vi "laneleftright.vi"() -> (2 "Coeff right":dbl[](array[numeric]), 3 "Coeff left":dbl[](array[numeric]))   [LabVIEW 2015]
uses:
  G_LCM.vi
  G_SEN.vi
  <vilib>/Analysis/1siggen.llb/Ramp Pattern by Delta.vi
  <vilib>/Analysis/polynomials.llb/1D Polynomial Evaluation (DBL).vi
  <vilib>/Analysis/NI_AALPro.lvlib
  <vilib>/Analysis/NI_AALBase.lvlib
panel:
  out "c_tmp":dbl[](array[numeric])
  out "y_tmp":dbl[](array[numeric])
  out "x_tmp":dbl[](array[numeric])
  out "Boolean":bool
  out "y origin":dbl[](array[numeric])
  out "x origin":dbl[](array[numeric])
  out "Histogram Graph 2":T1(graph)
  out "right":dbl[](graph)
  out "left":dbl[](graph)
  in  "Numeric":i32=4
  out "error left":dbl[](array[numeric])
  out "error right":dbl[](array[numeric])
  out "y seed":dbl[](array[numeric])
  out "XY Graph 4":cluster{"Y":dbl[], "Y":dbl[]}[](graph)=[{"Y"=array[3210 elements], "Y"=array[3210 elements]}, {"Y"=[-0.0, 0.001154394197769193, 0.004617650635850623, 0.010389990872226917, 0.018471784248973222, 0.02886354801042046, 0.041565947468740205, 0.056579796217107514, 0.0739060563904701, 0.0935458389742223, 0.11550040416098284, 0.13977116175580306, 0.16635967162997645, 0.19526764422393228, 0.2264969410994837, 0.26004957554195585, 0.2959277132125635, 0.3341336728515216, 0.374669927032528, 0.417539102969144, 0.4627439833735707, 0.5102875073687159, 0.560172771454063, 0.6124030305261954, 0.6669816989546717, 0.7239123517142048, 0.7831987255740245, 0.8448447203451934, 0.9088544001870815, 0.975231994973953, 1.0439819017227023, 1.1151086860829622, 1.1886170838907617, 1.2645120027869723, 1.342798523901962, 1.42348190360768, 1.5065675753387922, 1.592061151484188, 1.6799684253507792, 1.770295373200753, 1.8630481563645134, 1.9582331234307588, 2.0558568125157564, 2.1559259536137603, 2.258447471030621], "Y"=[0.0, 0.5, 1.0, 1.5, 2.0, 2.5, 3.0, 3.5, 4.0, 4.5, 5.0, 5.5, 6.0, 6.5, 7.0, 7.5, 8.0, 8.5, 9.0, 9.5, 10.0, 10.5, 11.0, 11.5, 12.0, 12.5, 13.0, 13.5, 14.0, 14.5, 15.0, 15.5, 16.0, 16.5, 17.0, 17.5, 18.0, 18.5, 19.0, 19.5, 20.0, 20.5, 21.0, 21.5, 22.0]}, {"Y"=[0.362252581831572], "Y"=[-0.8199241909738847]}, {"Y"=array[210 elements], "Y"=array[210 elements]}, {"Y"=[-0.925, -0.925, -0.925, -0.6775, -0.6775, -0.925, -0.925, -0.925, -0.925, -0.6775, -0.6775, -0.925, -0.925, -0.925, 0.9025, 0.9025, 0.9025, 0.6775, 0.6775, 0.9025, 0.9025, 0.9025, 0.9025, 0.6775, 0.6775, 0.9025, 0.9025, 0.9025, -0.925], "Y"=[-0.75, -0.224, 0.224, 0.224, -0.224, -0.224, 0.224, 2.415, 2.885, 2.885, 2.415, 2.415, 2.885, 3.5, 3.5, 2.885, 2.415, 2.415, 2.885, 2.885, 2.415, 0.224, -0.224, -0.224, 0.224, 0.224, -0.224, -0.75, -0.75]}, {"Y"=[0.171875, 0.15377271904051304, 0.1346290179491043, 0.11445423440635205, 0.09325870609283447, 0.07105277068912982, 0.04784676587581635, 0.02365102933347224, -0.0015241012573242174, -0.02766828821599482, -0.05477119386196136, -0.08282248051464558, -0.11181181049346922, -0.14172884611785413, -0.17256324970722198, -0.20430468358099463, -0.23694281005859374, -0.27046729145944115, -0.30486779010295867, -0.340133968308568, -0.3762554883956909, -0.41322201268374914, -0.4510232034921646, -0.4896487231403589], "Y"=[0.0, 0.5, 1.0, 1.5, 2.0, 2.5, 3.0, 3.5, 4.0, 4.5, 5.0, 5.5, 6.0, 6.5, 7.0, 7.5, 8.0, 8.5, 9.0, 9.5, 10.0, 10.5, 11.0, 11.5]}, {"Y"=[1.796875, 1.778772719040513, 1.7596290179491043, 1.739454234406352, 1.7182587060928345, 1.6960527706891297, 1.6728467658758164, 1.6486510293334722, 1.6234758987426758, 1.5973317117840051, 1.5702288061380387, 1.5421775194853544, 1.513188189506531, 1.483271153882146, 1.452436750292778, 1.4206953164190055, 1.3880571899414063, 1.354532708540559, 1.3201322098970414, 1.284866031691432, 1.248744511604309, 1.2117779873162509, 1.1739767965078354, 1.135351276859641, 1.0959117660522462, 1.0556686017662287, 1.014632121682167, 0.9728126634806396, 0.9302205648422242, 0.8868661634474992], "Y"=[0.0, 0.5, 1.0, 1.5, 2.0, 2.5, 3.0, 3.5, 4.0, 4.5, 5.0, 5.5, 6.0, 6.5, 7.0, 7.5, 8.0, 8.5, 9.0, 9.5, 10.0, 10.5, 11.0, 11.5, 12.0, 12.5, 13.0, 13.5, 14.0, 14.5]}, {"Y"=[-1.453125, -1.471227280959487, -1.4903709820508957, -1.510545765593648, -1.5317412939071655, -1.5539472293108703, -1.5771532341241836, -1.6013489706665278, -1.6265241012573242, -1.6526682882159949, -1.6797711938619613, -1.7078224805146456, -1.736811810493469, -1.766728846117854, -1.797563249707222, -1.8293046835809945, -1.8619428100585937, -1.895467291459441, -1.9298677901029586], "Y"=[0.0, 0.5, 1.0, 1.5, 2.0, 2.5, 3.0, 3.5, 4.0, 4.5, 5.0, 5.5, 6.0, 6.5, 7.0, 7.5, 8.0, 8.5, 9.0]}, {"Y"=[0.171875, 0.2568230007600336, 0.3384052130063493, 0.44574342526006827, 0.5205081969556753, 0.5917680690742042, 0.659409530134929, 0.7229937549325056, 0.7835496148685115, 0.8405449546633443, 0.9258576868463875], "Y"=[-20.239964538708662, -19.725637940364884, -19.211158961966362, -18.6998967366845, -18.19022720070031, -17.681887266143153, -17.17615515566314, -16.67683575591291, -16.176265245349786, -15.679082775270938, -15.183754484614711]}, {"Y"=[7.134647485270904], "Y"=[38.71960961082238]}, {"Y"=array[980 elements], "Y"=array[980 elements]}, {"Y"=[], "Y"=[]}]
  out "y all":dbl[](array[numeric])
  out "x all":dbl[](array[numeric])
  out "x_left":dbl[](array[numeric])
  out "x_right":dbl[](array[numeric])
  out "y_left":dbl[](array[numeric])
  out "y_right":dbl[](array[numeric])
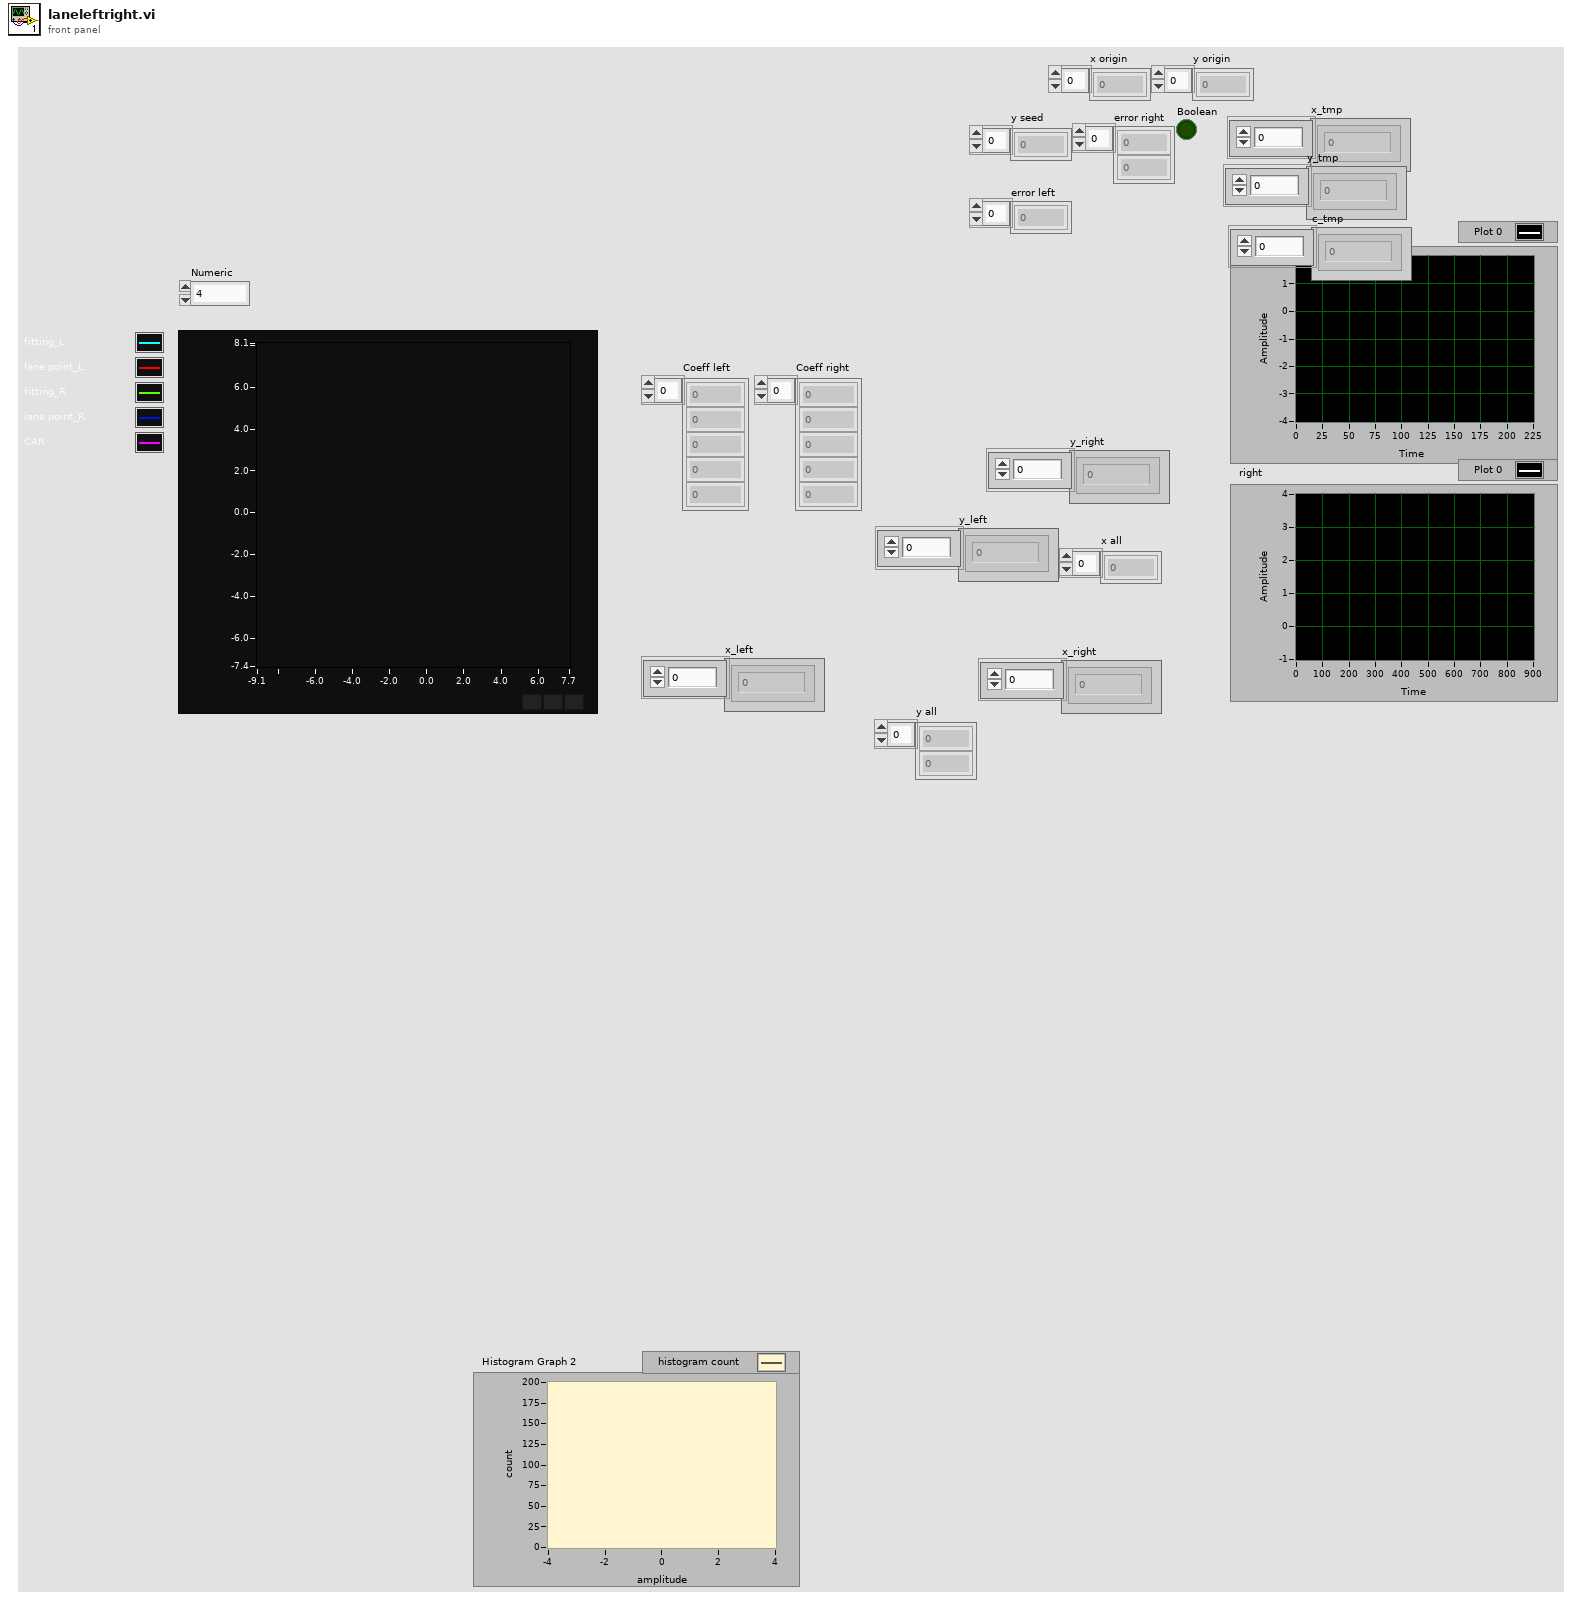
[diagram p1: front panel]
types:
  T1 = cluster{"X Values":dbl[], "Histogram: h(x)":i32[]}
  T2 = cluster{"hash":i64, "sys time":i64, "size":i64, "x":dbl[], "y":dbl[]}
  T3 = cluster{"delta":bool, "Rotational position":dbl, "Rotational position":dbl}[]
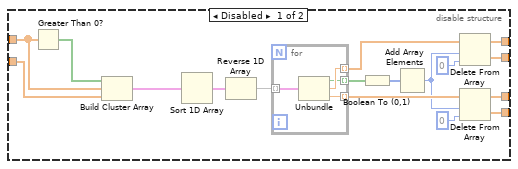
[diagram p3: hidden frame]
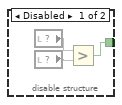
[diagram p6: hidden frame]
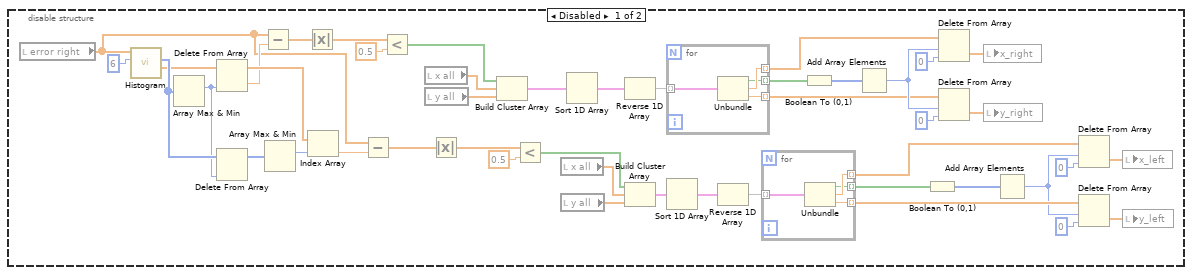
[diagram p7: hidden frame]
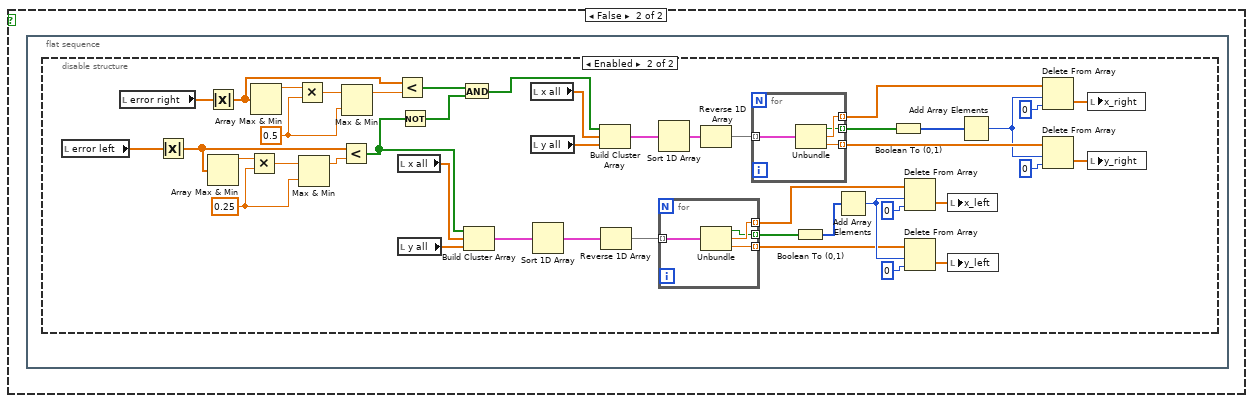
[diagram p8: hidden frame]
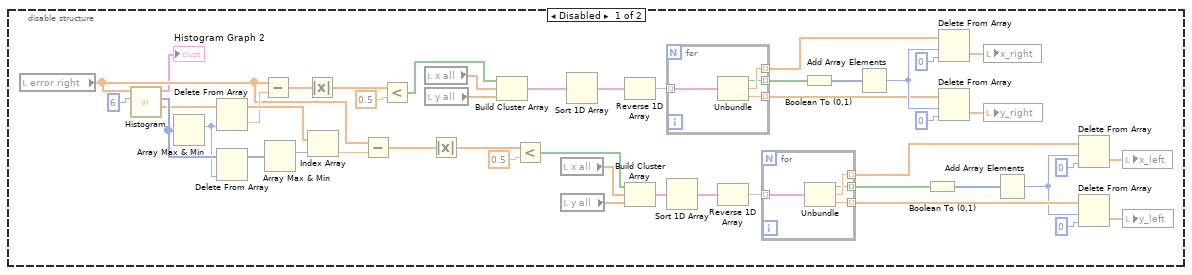
[diagram p9: hidden frame]
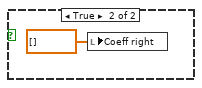
[diagram p12: hidden frame]
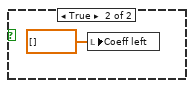
[diagram p13: hidden frame]
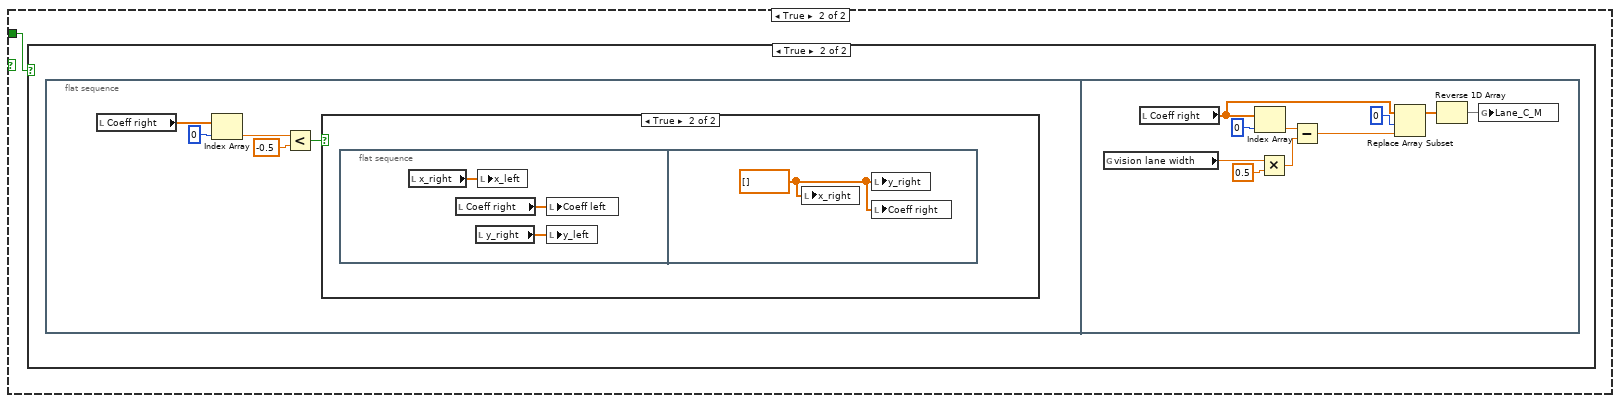
[diagram p15: hidden frame]
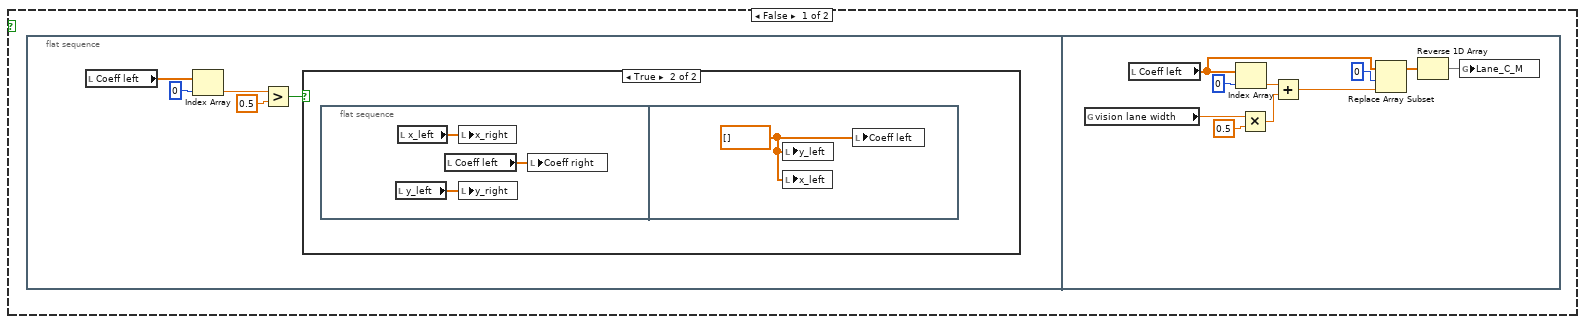
[diagram p16: hidden frame]
diagram:
  n1 = flat-sequence {
    frame #0 {
      n2 = global read "G_LCM.vi" "VISION_LANE_PT"() -> (w20:T2)
      n3 = First Call?() -> (First Call?: T/F=w1:bool)
      n4 = case shown="True" w1 {
        frame False {
        }
        frame True {
          n5 = global write "G_SEN.vi" "vision lane width"(3.5 ("vision lane width")) -> ()
          n6 = call-poly <vilib>:"Ramp Pattern.vi"("start"=-4.0, "end"=6.0, "delta"=0.1) -> ("Ramp Pattern"=w24:dbl[])  [unwired: 6 in, 2 out]
          n7 = global write "G_SEN.vi" "y_mobileye"(w24) -> ()
        }
      }
      n8 = Unbundle By Name(w20) -> ("y"=w19:dbl[], "x"=w16:dbl[], "y"=w3:dbl[])
      "x origin" <- w16
      "y origin" <- w3
      n9 = In Range and Coerce(upper limit=5.0 ("delta"), x=w19, lower limit=-4.0) -> (In Range?=w17:bool[])  [unwired: 1 out]
      n10 = Build Cluster Array(w17, w16, w3) -> (w14:T3)
      n11 = Sort 1D Array(array=w14) -> (sorted array=w15:T3)
      n12 = Reverse 1D Array(array=w15) -> (reversed array=w6:T3)
      n13 = for {
        tunnel: w6 -> [w29] mode=indexing
        tunnel: [w28] -> w9 mode=indexing
        tunnel: [w27] -> w10 mode=indexing
        tunnel: [w26] -> w7 mode=indexing
        n14 = Unbundle(w29) -> ("delta"=w26:bool, "Rotational position"=w28:dbl, "Rotational position"=w27:dbl)
      }
      n15 = Boolean To (0,1)(Boolean=w7) -> (0, 1=w8:i16[])
      n16 = Add Array Elements(numeric array=w8) -> (sum=w11:i16)
      n17 = Delete From Array(array=w9, length=w11, index=0) -> (deleted portion=→"x all":dbl[])  [unwired: 1 out]
      n18 = Delete From Array(array=w10, length=w11, index=0) -> (deleted portion=→"y all":dbl[])  [unwired: 1 out]
    }
    frame #1 {
      n19 = local read "x all"() -> (w31:dbl[])
      n20 = local read "y all"() -> (w30:dbl[])
      n21 = disable-structure shown="Enabled" {
        disable-tunnel: w31 -> [w41 w62]
        disable-tunnel: w30 -> [w52 w61]
        disable-tunnel: [w39 w66] -> w32
        disable-tunnel: [w38 w65] -> w35
        disable-tunnel: [w37 w64] -> w34
        disable-tunnel: [w36 w63] -> w33
        frame Disabled {
          n22 = Greater Than 0?(x=w41) -> (x > 0?=w40:bool[])
          n23 = Build Cluster Array(w40, w41, w52) -> (w51:cluster{bool, dbl, dbl}[])
          n24 = Sort 1D Array(array=w51) -> (sorted array=w50:cluster{bool, dbl, dbl}[])
          n25 = Reverse 1D Array(array=w50) -> (reversed array=w49:cluster{bool, dbl, dbl}[])
          n26 = for {
            tunnel: w49 -> [w56] mode=indexing
            tunnel: [w55] -> w46 mode=indexing
            tunnel: [w54] -> w45 mode=indexing
            tunnel: [w53] -> w48 mode=indexing
            n27 = Unbundle(w56) -> (w53:bool, w55:dbl, w54:dbl)
          }
          n28 = Boolean To (0,1)(Boolean=w48) -> (0, 1=w47:i16[])
          n29 = Add Array Elements(numeric array=w47) -> (sum=w44:i16)
          n30 = Delete From Array(array=w46, length=w44, index=0) -> (deleted portion=w38:dbl[], array with subset deleted=w39:dbl[])
          n31 = Delete From Array(array=w45, length=w44, index=0) -> (deleted portion=w36:dbl[], array with subset deleted=w37:dbl[])
        }
        frame Enabled {
          n32 = Greater Than 0?(x=w62) -> (x > 0?=w67:bool[])
          n33 = Array Max & Min(array=w61) -> (max value=w60:dbl, min value=w59:dbl)  [unwired: 2 out]
          n34 = Build Cluster Array(w67, w62, w61) -> (w77:cluster{bool, dbl, dbl}[])
          n35 = call-poly <vilib>:"Ramp Pattern.vi"("start"=w59, "end"=w60, "delta"=0.01) -> ("Ramp Pattern"=→"y seed":dbl[])  [unwired: 6 in, 2 out]
          n36 = Sort 1D Array(array=w77) -> (sorted array=w76:cluster{bool, dbl, dbl}[])
          n37 = Reverse 1D Array(array=w76) -> (reversed array=w75:cluster{bool, dbl, dbl}[])
          n38 = for {
            tunnel: w75 -> [w81] mode=indexing
            tunnel: [w80] -> w72 mode=indexing
            tunnel: [w79] -> w71 mode=indexing
            tunnel: [w78] -> w74 mode=indexing
            n39 = Unbundle(w81) -> (w78:bool, w80:dbl, w79:dbl)
          }
          n40 = Boolean To (0,1)(Boolean=w74) -> (0, 1=w73:i16[])
          n41 = Add Array Elements(numeric array=w73) -> (sum=w70:i16)
          n42 = Delete From Array(array=w72, length=w70, index=0) -> (deleted portion=w65:dbl[], array with subset deleted=w66:dbl[])
          n43 = Delete From Array(array=w71, length=w70, index=0) -> (deleted portion=w63:dbl[], array with subset deleted=w64:dbl[])
        }
      }
      "x_left" <- w32
      "x_right" <- w35
      "y_left" <- w34
      "y_right" <- w33
    }
    frame #2 {
      n44 = disable-structure shown="Enabled" {
        frame Enabled {
          n45 = local read "x_left"() -> (w83:dbl[])
          n46 = Array Size(array=w83) -> (size(s)=w82:i32)
          n47 = for {
            N: w82 -> [_]
            tunnel: [w95] -> w85 mode=indexing
            tunnel: [w88] -> w84 mode=indexing
            i -> [w88]
            n48 = local read "x_left"() -> (w89:dbl[])
            n49 = local read "y_left"() -> (w92:dbl[])
            n50 = Build Array(w89, w92) -> (w91:dbl[][])
            n51 = Index Array(array=w91, index (col)=w88) -> (element=w90:dbl[])  [unwired: 1 in]
            n52 = Build Array(0.0 ("element"), 0.0 ("element")) -> (w98:dbl[])
            n53 = Subtract(x=w90, y=w98) -> (x-y=w99:dbl[])
            n54 = Square(x=w99) -> (x^2=w100:dbl[])
            n55 = Index Array(array=w100, index #1=0 ("index"), index #2=1 ("index")) -> (element #1=w102:dbl, element #2=w103:dbl)
            n56 = Add(x=w102, y=w103) -> (x+y=w96:dbl)
            n57 = Less Or Equal?(x=w96, y=36.0) -> (x <= y?=w95:bool)
          }
          n58 = Or Array Elements(Boolean array=w85) -> (logical OR=w86:bool)
          n59 = case shown="True" w86 {
            tunnel: w84 -> [_ w87]
            frame False {
            }
            frame True {
              n60 = Array Max & Min(array=w87) -> ()  [unwired: 4 out]
            }
          }
        }
        frame Disabled {
        }
      }
    }
    frame #3 {
      n61 = for {
        N: "Numeric" -> [_]
        stop <- w106 stop-if-true
        n62 = flat-sequence {
          tunnel: [w390] -> w106
          frame #0 {
            n63 = local read "x_left"() -> (w114:dbl[])
            n64 = Negate(x=w114) -> (-x=w116:dbl[])
            n65 = local read "y_left"() -> (w115:dbl[])
            n66 = call <vilib>:"General Polynomial Fit Coefficients.vi"("Y"=w116, "polynomial order"=2, "X"=w115) -> ("Polynomial Coefficients"=w110:dbl[])  [unwired: 11 in, 1 out]
            n67 = Negate(x=w110) -> (-x=w108:dbl[])
            "Coeff left" <- w108
            n68 = local read "y all"() -> (w113:dbl[])
            n69 = call-poly <vilib>:"Polynomial Evaluation.vi"("P(x)"=w108, "A"=w113) -> ("P(A)"=w112:dbl[])  [unwired: 1 out]
            n70 = local read "x all"() -> (w111:dbl[])
            n71 = Subtract(x=w112, y=w111) -> (x-y=→"error left":dbl[])
          }
          frame #1 {
            n72 = local read "x_right"() -> (w124:dbl[])
            n73 = local read "y_right"() -> (w120:dbl[])
            n74 = Negate(x=w124) -> (-x=w125:dbl[])
            n75 = call <vilib>:"General Polynomial Fit Coefficients.vi"("Y"=w125, "polynomial order"=2, "X"=w120) -> ("Polynomial Coefficients"=w119:dbl[])  [unwired: 11 in, 1 out]
            n76 = Negate(x=w119) -> (-x=w118:dbl[])
            "Coeff right" <- w118
            n77 = local read "y all"() -> (w121:dbl[])
            n78 = call-poly <vilib>:"Polynomial Evaluation.vi"("P(x)"=w118, "A"=w121) -> ("P(A)"=w122:dbl[])  [unwired: 1 out]
            n79 = local read "x all"() -> (w123:dbl[])
            n80 = Subtract(x=w122, y=w123) -> (x-y=→"error right":dbl[])
          }
          frame #2 {
            n81 = disable-structure shown="Enabled" {
              disable-tunnel: [w128 w133] -> w127
              frame Disabled {
                n82 = local read item#-1() -> (w129)
                n83 = local read item#-1() -> (w130)
                n84 = Greater?(x=w129, y=w130) -> (0:w128:bool)
              }
              frame Enabled {
                n85 = local read "error right"() -> (w167:dbl[])
                n86 = local read "error left"() -> (w166:dbl[])
                n87 = local read "Coeff right"() -> (w147:dbl[])
                n88 = local read "Coeff left"() -> (w136:dbl[])
                n89 = call <vilib>:"General Histogram.vi"("X"=w166) -> ("Histogram"=w163:i32[])  [unwired: 10 in, 4 out]
                n90 = call <vilib>:"General Histogram.vi"("X"=w167) -> ("Histogram"=w150:i32[])  [unwired: 10 in, 4 out]
                n91 = Add Array Elements(numeric array=w163) -> (sum=w162:i32)
                n92 = Add Array Elements(numeric array=w150) -> (sum=w153:i32)
                n93 = Square(x=w163) -> (x^2=w165:i32[])
                n94 = Square(x=w150) -> (x^2=w151:i32[])
                n95 = Array Size(array=w163) -> (size(s)=w161:i32)
                n96 = Array Size(array=w150) -> (size(s)=w154:i32)
                n97 = Array Subset(array=w136, index=1) -> (w138:dbl[])  [unwired: 1 in]
                n98 = Array Subset(array=w147, index=1) -> (w145:dbl[])  [unwired: 1 in]
                n99 = Absolute Value(x=w138) -> (abs(x)=w139:dbl[])
                n100 = Absolute Value(x=w145) -> (abs(x)=w144:dbl[])
                n101 = Add Array Elements(numeric array=w165) -> (sum=w164:i32)
                n102 = Divide(x=w162, y=w161) -> (x/y=w159:dbl)
                n103 = Add Array Elements(numeric array=w151) -> (sum=w152:i32)
                n104 = Divide(x=w153, y=w154) -> (x/y=w156:dbl)
                n105 = Divide(x=w164, y=w161) -> (x/y=w160:dbl)
                n106 = Divide(x=w152, y=w154) -> (x/y=w155:dbl)
                n107 = Square(x=w159) -> (x^2=w158:dbl)
                n108 = Square(x=w156) -> (x^2=w157:dbl)
                n109 = Greater?(x=w139, y=1.0) -> (0:w141:bool[])
                n110 = Greater?(x=w144, y=1.0) -> (0:w142:bool[])
                n111 = Or Array Elements(Boolean array=w141) -> (logical OR=w132:bool)
                n112 = Or Array Elements(Boolean array=w142) -> (logical OR=w131:bool)
                n113 = Subtract(x=w160, y=w158) -> (x-y=w149:dbl)
                n114 = Subtract(x=w155, y=w157) -> (x-y=w148:dbl)
                n115 = Less?(x=w149, y=w148) -> (x < y?=w134:bool)
                n116 = Exclusive Or(1:w131, 2:w132) -> (0:w135:bool)
                n117 = Select(t=w132, s=w135, f=w134) -> (s? t:f=w133:bool)
              }
            }
            "Boolean" <- w127
            n118 = case shown="True" w127 {
              frame True {
                n119 = flat-sequence {
                  frame #0 {
                    n120 = disable-structure shown="Enabled" {
                      frame Disabled {
                        n121 = local read "error right"() -> (w170:dbl[])
                        n122 = call <vilib>:"Histogram.vi"("intervals"=6, "X"=w170) -> ("X Values"=w212:dbl[], "Histogram: h(x)"=w214:i32[], "Histogram Graph"=w168:T1)  [unwired: 6 in, 1 out]
                        n123 = Array Max & Min(array=w214) -> (max index (indices)=w211:i32)  [unwired: 3 out]
                        n124 = Delete From Array(array=w212, index=w211) -> (deleted portion=w208:dbl, array with subset deleted=w210:dbl[])  [unwired: 1 in]
                        n125 = Delete From Array(array=w214, index=w211) -> (array with subset deleted=w213:i32[])  [unwired: 1 in, 1 out]
                        n126 = Subtract(x=w170, y=w208) -> (x-y=w172:dbl[])
                        n127 = Array Max & Min(array=w213) -> (max index (indices)=w209:i32)  [unwired: 3 out]
                        n128 = Absolute Value(x=w172) -> (abs(x)=w171:dbl[])
                        n129 = Index Array(array=w210, index=w209) -> (element=w190:dbl)
                        n130 = Subtract(x=w170, y=w190) -> (x-y=w174:dbl[])
                        n131 = Less?(x=w171, y=0.5) -> (x < y?=w192:bool[])
                        n132 = local read "x all"() -> (w203:dbl[])
                        n133 = local read "y all"() -> (w204:dbl[])
                        n134 = Absolute Value(x=w174) -> (abs(x)=w173:dbl[])
                        n135 = Build Cluster Array(w192, w203, w204) -> (w193:cluster{bool, dbl, dbl}[])
                        n136 = Less?(x=w173, y=0.5) -> (x < y?=w175:bool[])
                        n137 = local read "x all"() -> (w179:dbl[])
                        n138 = local read "y all"() -> (w178:dbl[])
                        n139 = Sort 1D Array(array=w193) -> (sorted array=w194:cluster{bool, dbl, dbl}[])
                        n140 = Reverse 1D Array(array=w194) -> (reversed array=w195:cluster{bool, dbl, dbl}[])
                        n141 = Build Cluster Array(w175, w179, w178) -> (w189:cluster{bool, dbl, dbl}[])
                        n142 = for {
                          tunnel: w195 -> [w222] mode=indexing
                          tunnel: [w221] -> w198 mode=indexing
                          tunnel: [w220] -> w199 mode=indexing
                          tunnel: [w219] -> w196 mode=indexing
                          n143 = Unbundle(w222) -> (w219:bool, w221:dbl, w220:dbl)
                        }
                        n144 = Sort 1D Array(array=w189) -> (sorted array=w188:cluster{bool, dbl, dbl}[])
                        n145 = Reverse 1D Array(array=w188) -> (reversed array=w187:cluster{bool, dbl, dbl}[])
                        n146 = for {
                          tunnel: w187 -> [w218] mode=indexing
                          tunnel: [w217] -> w184 mode=indexing
                          tunnel: [w216] -> w183 mode=indexing
                          tunnel: [w215] -> w186 mode=indexing
                          n147 = Unbundle(w218) -> (w215:bool, w217:dbl, w216:dbl)
                        }
                        n148 = Boolean To (0,1)(Boolean=w196) -> (0, 1=w197:i16[])
                        n149 = Add Array Elements(numeric array=w197) -> (sum=w200:i16)
                        n150 = Boolean To (0,1)(Boolean=w186) -> (0, 1=w185:i16[])
                        n151 = Delete From Array(array=w198, length=w200, index=0) -> (deleted portion=w205:dbl[])  [unwired: 1 out]
                        n152 = Delete From Array(array=w199, length=w200, index=0) -> (deleted portion=w206:dbl[])  [unwired: 1 out]
                        n153 = local write "x_right"(w205) -> ()
                        n154 = local write "y_right"(w206) -> ()
                        n155 = Add Array Elements(numeric array=w185) -> (sum=w182:i16)
                        n156 = Delete From Array(array=w184, length=w182, index=0) -> (deleted portion=w177:dbl[])  [unwired: 1 out]
                        n157 = Delete From Array(array=w183, length=w182, index=0) -> (deleted portion=w176:dbl[])  [unwired: 1 out]
                        n158 = local write "x_left"(w177) -> ()
                        n159 = local write "y_left"(w176) -> ()
                      }
                      frame Enabled {
                        w223 = 0.5 ("y")
                        w227 = 0.25 ("y")
                        n160 = local read "error right"() -> (w265:dbl[])
                        n161 = local read "error left"() -> (w236:dbl[])
                        n162 = Absolute Value(x=w265) -> (abs(x)=w229:dbl[])
                        n163 = Array Max & Min(array=w229) -> (max value=w266:dbl)  [unwired: 3 out]
                        n164 = Absolute Value(x=w236) -> (abs(x)=w230:dbl[])
                        n165 = Multiply(x=w266, y=w227) -> (x*y=w228:dbl)
                        n166 = Array Max & Min(array=w230) -> (max value=w235:dbl)  [unwired: 3 out]
                        n167 = Multiply(x=w235, y=w223) -> (x*y=w225:dbl)
                        n168 = Max & Min(x=w228, y=w227) -> (max(x,y)=w226:dbl)  [unwired: 1 out]
                        n169 = Less?(x=w229, y=w226) -> (x < y?=w234:bool[])
                        n170 = Max & Min(x=w225, y=w223) -> (max(x,y)=w224:dbl)  [unwired: 1 out]
                        n171 = Less?(x=w230, y=w224) -> (x < y?=w231:bool[])
                        n172 = local read "x all"() -> (w261:dbl[])
                        n173 = local read "y all"() -> (w262:dbl[])
                        n174 = Not(x=w234) -> (.not. x?=w233:bool[])
                        n175 = And(x=w233, y=w231) -> (x .and. y?=w232:bool[])
                        n176 = Build Cluster Array(w234, w261, w262) -> (w251:cluster{bool, dbl, dbl}[])
                        n177 = local read "x all"() -> (w240:dbl[])
                        n178 = local read "y all"() -> (w239:dbl[])
                        n179 = Sort 1D Array(array=w251) -> (sorted array=w252:cluster{bool, dbl, dbl}[])
                        n180 = Build Cluster Array(w232, w240, w239) -> (w250:cluster{bool, dbl, dbl}[])
                        n181 = Reverse 1D Array(array=w252) -> (reversed array=w253:cluster{bool, dbl, dbl}[])
                        n182 = for {
                          tunnel: w253 -> [w274] mode=indexing
                          tunnel: [w273] -> w256 mode=indexing
                          tunnel: [w272] -> w257 mode=indexing
                          tunnel: [w271] -> w254 mode=indexing
                          n183 = Unbundle(w274) -> (w271:bool, w273:dbl, w272:dbl)
                        }
                        n184 = Sort 1D Array(array=w250) -> (sorted array=w249:cluster{bool, dbl, dbl}[])
                        n185 = Reverse 1D Array(array=w249) -> (reversed array=w248:cluster{bool, dbl, dbl}[])
                        n186 = for {
                          tunnel: w248 -> [w270] mode=indexing
                          tunnel: [w269] -> w245 mode=indexing
                          tunnel: [w268] -> w244 mode=indexing
                          tunnel: [w267] -> w247 mode=indexing
                          n187 = Unbundle(w270) -> (w267:bool, w269:dbl, w268:dbl)
                        }
                        n188 = Boolean To (0,1)(Boolean=w254) -> (0, 1=w255:i16[])
                        n189 = Add Array Elements(numeric array=w255) -> (sum=w258:i16)
                        n190 = Boolean To (0,1)(Boolean=w247) -> (0, 1=w246:i16[])
                        n191 = Delete From Array(array=w256, length=w258, index=0) -> (deleted portion=w263:dbl[])  [unwired: 1 out]
                        n192 = Delete From Array(array=w257, length=w258, index=0) -> (deleted portion=w264:dbl[])  [unwired: 1 out]
                        n193 = local write "x_right"(w263) -> ()
                        n194 = local write "y_right"(w264) -> ()
                        n195 = Add Array Elements(numeric array=w246) -> (sum=w243:i16)
                        n196 = Delete From Array(array=w245, length=w243, index=0) -> (deleted portion=w238:dbl[])  [unwired: 1 out]
                        n197 = Delete From Array(array=w244, length=w243, index=0) -> (deleted portion=w237:dbl[])  [unwired: 1 out]
                        n198 = local write "x_left"(w238) -> ()
                        n199 = local write "y_left"(w237) -> ()
                      }
                    }
                  }
                }
              }
              frame False {
                n200 = flat-sequence {
                  frame #0 {
                    n201 = disable-structure shown="Enabled" {
                      frame Disabled {
                        n202 = local read "error right"() -> (w277:dbl[])
                        n203 = call <vilib>:"Histogram.vi"("intervals"=6, "X"=w277) -> ("X Values"=w319:dbl[], "Histogram: h(x)"=w321:i32[], "Histogram Graph"=→"Histogram Graph 2":T1)  [unwired: 6 in, 1 out]
                        n204 = Array Max & Min(array=w321) -> (max index (indices)=w318:i32)  [unwired: 3 out]
                        n205 = Delete From Array(array=w319, index=w318) -> (deleted portion=w315:dbl, array with subset deleted=w317:dbl[])  [unwired: 1 in]
                        n206 = Delete From Array(array=w321, index=w318) -> (array with subset deleted=w320:i32[])  [unwired: 1 in, 1 out]
                        n207 = Subtract(x=w277, y=w315) -> (x-y=w279:dbl[])
                        n208 = Array Max & Min(array=w320) -> (max index (indices)=w316:i32)  [unwired: 3 out]
                        n209 = Absolute Value(x=w279) -> (abs(x)=w278:dbl[])
                        n210 = Index Array(array=w317, index=w316) -> (element=w297:dbl)
                        n211 = Subtract(x=w277, y=w297) -> (x-y=w281:dbl[])
                        n212 = Less?(x=w278, y=0.5) -> (x < y?=w299:bool[])
                        n213 = local read "x all"() -> (w310:dbl[])
                        n214 = local read "y all"() -> (w311:dbl[])
                        n215 = Absolute Value(x=w281) -> (abs(x)=w280:dbl[])
                        n216 = Build Cluster Array(w299, w310, w311) -> (w300:cluster{bool, dbl, dbl}[])
                        n217 = Less?(x=w280, y=0.5) -> (x < y?=w282:bool[])
                        n218 = local read "x all"() -> (w286:dbl[])
                        n219 = local read "y all"() -> (w285:dbl[])
                        n220 = Sort 1D Array(array=w300) -> (sorted array=w301:cluster{bool, dbl, dbl}[])
                        n221 = Reverse 1D Array(array=w301) -> (reversed array=w302:cluster{bool, dbl, dbl}[])
                        n222 = Build Cluster Array(w282, w286, w285) -> (w296:cluster{bool, dbl, dbl}[])
                        n223 = for {
                          tunnel: w302 -> [w329] mode=indexing
                          tunnel: [w328] -> w305 mode=indexing
                          tunnel: [w327] -> w306 mode=indexing
                          tunnel: [w326] -> w303 mode=indexing
                          n224 = Unbundle(w329) -> (w326:bool, w328:dbl, w327:dbl)
                        }
                        n225 = Sort 1D Array(array=w296) -> (sorted array=w295:cluster{bool, dbl, dbl}[])
                        n226 = Reverse 1D Array(array=w295) -> (reversed array=w294:cluster{bool, dbl, dbl}[])
                        n227 = for {
                          tunnel: w294 -> [w325] mode=indexing
                          tunnel: [w324] -> w291 mode=indexing
                          tunnel: [w323] -> w290 mode=indexing
                          tunnel: [w322] -> w293 mode=indexing
                          n228 = Unbundle(w325) -> (w322:bool, w324:dbl, w323:dbl)
                        }
                        n229 = Boolean To (0,1)(Boolean=w303) -> (0, 1=w304:i16[])
                        n230 = Add Array Elements(numeric array=w304) -> (sum=w307:i16)
                        n231 = Boolean To (0,1)(Boolean=w293) -> (0, 1=w292:i16[])
                        n232 = Delete From Array(array=w305, length=w307, index=0) -> (deleted portion=w312:dbl[])  [unwired: 1 out]
                        n233 = Delete From Array(array=w306, length=w307, index=0) -> (deleted portion=w313:dbl[])  [unwired: 1 out]
                        n234 = local write "x_right"(w312) -> ()
                        n235 = local write "y_right"(w313) -> ()
                        n236 = Add Array Elements(numeric array=w292) -> (sum=w289:i16)
                        n237 = Delete From Array(array=w291, length=w289, index=0) -> (deleted portion=w284:dbl[])  [unwired: 1 out]
                        n238 = Delete From Array(array=w290, length=w289, index=0) -> (deleted portion=w283:dbl[])  [unwired: 1 out]
                        n239 = local write "x_left"(w284) -> ()
                        n240 = local write "y_left"(w283) -> ()
                      }
                      frame Enabled {
                        w333 = 0.5 ("y")
                        w330 = 0.25 ("y")
                        n241 = local read "error left"() -> (w372:dbl[])
                        n242 = local read "error right"() -> (w343:dbl[])
                        n243 = Absolute Value(x=w372) -> (abs(x)=w338:dbl[])
                        n244 = Absolute Value(x=w343) -> (abs(x)=w339:dbl[])
                        n245 = Array Max & Min(array=w338) -> (max value=w373:dbl)  [unwired: 3 out]
                        n246 = Multiply(x=w373, y=w330) -> (x*y=w337:dbl)
                        n247 = Array Max & Min(array=w339) -> (max value=w342:dbl)  [unwired: 3 out]
                        n248 = Multiply(x=w342, y=w333) -> (x*y=w335:dbl)
                        n249 = Max & Min(x=w337, y=w330) -> (max(x,y)=w336:dbl)  [unwired: 1 out]
                        n250 = Less?(x=w338, y=w336) -> (x < y?=w341:bool[])
                        n251 = Max & Min(x=w335, y=w333) -> (max(x,y)=w334:dbl)  [unwired: 1 out]
                        n252 = Less?(x=w339, y=w334) -> (x < y?=w332:bool[])
                        n253 = local read "x all"() -> (w368:dbl[])
                        n254 = local read "y all"() -> (w369:dbl[])
                        n255 = Not(x=w341) -> (.not. x?=w331:bool[])
                        n256 = And(x=w332, y=w331) -> (x .and. y?=w340:bool[])
                        n257 = Build Cluster Array(w341, w368, w369) -> (w358:cluster{bool, dbl, dbl}[])
                        n258 = local read "x all"() -> (w347:dbl[])
                        n259 = local read "y all"() -> (w346:dbl[])
                        n260 = Sort 1D Array(array=w358) -> (sorted array=w359:cluster{bool, dbl, dbl}[])
                        n261 = Build Cluster Array(w340, w347, w346) -> (w357:cluster{bool, dbl, dbl}[])
                        n262 = Reverse 1D Array(array=w359) -> (reversed array=w360:cluster{bool, dbl, dbl}[])
                        n263 = Sort 1D Array(array=w357) -> (sorted array=w356:cluster{bool, dbl, dbl}[])
                        n264 = for {
                          tunnel: w360 -> [w381] mode=indexing
                          tunnel: [w380] -> w363 mode=indexing
                          tunnel: [w379] -> w364 mode=indexing
                          tunnel: [w378] -> w361 mode=indexing
                          n265 = Unbundle(w381) -> (w378:bool, w380:dbl, w379:dbl)
                        }
                        n266 = Reverse 1D Array(array=w356) -> (reversed array=w355:cluster{bool, dbl, dbl}[])
                        n267 = for {
                          tunnel: w355 -> [w377] mode=indexing
                          tunnel: [w376] -> w352 mode=indexing
                          tunnel: [w375] -> w351 mode=indexing
                          tunnel: [w374] -> w354 mode=indexing
                          n268 = Unbundle(w377) -> (w374:bool, w376:dbl, w375:dbl)
                        }
                        n269 = Boolean To (0,1)(Boolean=w361) -> (0, 1=w362:i16[])
                        n270 = Add Array Elements(numeric array=w362) -> (sum=w365:i16)
                        n271 = Boolean To (0,1)(Boolean=w354) -> (0, 1=w353:i16[])
                        n272 = Delete From Array(array=w363, length=w365, index=0) -> (deleted portion=w370:dbl[])  [unwired: 1 out]
                        n273 = Delete From Array(array=w364, length=w365, index=0) -> (deleted portion=w371:dbl[])  [unwired: 1 out]
                        n274 = local write "x_left"(w370) -> ()
                        n275 = local write "y_left"(w371) -> ()
                        n276 = Add Array Elements(numeric array=w353) -> (sum=w350:i16)
                        n277 = Delete From Array(array=w352, length=w350, index=0) -> (deleted portion=w345:dbl[])  [unwired: 1 out]
                        n278 = Delete From Array(array=w351, length=w350, index=0) -> (deleted portion=w344:dbl[])  [unwired: 1 out]
                        n279 = local write "x_right"(w345) -> ()
                        n280 = local write "y_right"(w344) -> ()
                      }
                    }
                  }
                }
              }
            }
          }
          frame #3 {
            n281 = local read "y_right"() -> (w389:dbl[])
            n282 = local read "y_left"() -> (w384:dbl[])
            n283 = Array Size(array=w389) -> (size(s)=w388:i32)
            n284 = Array Size(array=w384) -> (size(s)=w385:i32)
            n285 = Less?(x=w388, y=20) -> (x < y?=w383:bool)
            n286 = Less?(x=w385, y=20) -> (x < y?=w382:bool)
            n287 = Or(x=w383, y=w382) -> (x .or. y?=w390:bool)
            n288 = case shown="True" w383 {
              frame False {
              }
              frame True {
                n289 = local write "Coeff right"(dbl[] []) -> ()
              }
            }
            n290 = case shown="True" w382 {
              frame False {
              }
              frame True {
                n291 = local write "Coeff left"(dbl[] []) -> ()
              }
            }
          }
        }
      }
    }
    frame #4 {
      n292 = local read "y_right"() -> (w395:dbl[])
      n293 = Array Size(array=w395) -> (size(s)=w394:i32)
      n294 = Less?(x=w394, y=60) -> (x < y?=w396:bool)
      n295 = case shown="False" w396 {
        frame False {
          n296 = for {
            N: 3 -> [_]
            tunnel: [w417] -> w404 mode=indexing
            tunnel: [w414] -> w413 mode=indexing
            i -> [w416]
            n297 = local read "x_right"() -> (w426:dbl[])
            n298 = local read "y_right"() -> (w427:dbl[])
            n299 = Negate(x=w426) -> (-x=w428:dbl[])
            n300 = Increment(x=w416) -> (x+1=w415:i32)
            n301 = call <vilib>:"General Polynomial Fit Coefficients.vi"("Y"=w428, "polynomial order"=w415, "X"=w427) -> ("Polynomial Coefficients"=w424:dbl[])  [unwired: 11 in, 1 out]
            n302 = local read "y_right"() -> (w423:dbl[])
            n303 = Negate(x=w424) -> (-x=w414:dbl[])
            n304 = call-poly <vilib>:"Polynomial Evaluation.vi"("P(x)"=w414, "A"=w423) -> ("P(A)"=w425:dbl[])  [unwired: 1 out]
            n305 = local read "x_right"() -> (w422:dbl[])
            n306 = Subtract(x=w425, y=w422) -> (x-y=w419:dbl[])
            n307 = Absolute Value(x=w419) -> (abs(x)=w418:dbl[])
            n308 = Add Array Elements(numeric array=w418) -> (sum=w421:dbl)
            n309 = Array Size(array=w418) -> (size(s)=w420:i32)
            n310 = Divide(x=w421, y=w420) -> (x/y=w417:dbl)
          }
          n311 = Multiply(x=w404, y=dbl[] [1.0, 1.1, 1.15]) -> (x*y=w403:dbl[])
          n312 = Array Max & Min(array=w403) -> (min index (indices)=w401:i32)  [unwired: 3 out]
          n313 = Index Array(array=w413, index (row)=w401) -> (element=w398:dbl[])  [unwired: 1 in]
          n314 = Array Subset(array=w398, index=1) -> (w410:dbl[])  [unwired: 1 in]
          n315 = Absolute Value(x=w410) -> (abs(x)=w409:dbl[])
          n316 = Not Equal To 0?(x=w401) -> (x != 0?=w400:bool)
          n317 = Greater?(x=w409, y=1.0) -> (0:w407:bool[])
          n318 = Or Array Elements(Boolean array=w407) -> (logical OR=w406:bool)
          n319 = Select(t=dbl[] [], s=w406, f=w398) -> (s? t:f=w399:dbl[])
          n320 = Select(t=w399, s=w400, f=w398) -> (s? t:f=w397:dbl[])
          n321 = local write "Coeff right"(w397) -> ()
        }
        frame True {
          n322 = local write "Coeff right"(dbl[] []) -> ()
        }
      }
    }
    frame #5 {
      n323 = local read "y_left"() -> (w433:dbl[])
      n324 = Array Size(array=w433) -> (size(s)=w432:i32)
      n325 = Less?(x=w432, y=60) -> (x < y?=w430:bool)
      n326 = case shown="False" w430 {
        frame False {
          n327 = for {
            N: 3 -> [_]
            tunnel: [w454] -> w440 mode=indexing
            tunnel: [w451] -> w449 mode=indexing
            i -> [w453]
            n328 = local read "x_left"() -> (w463:dbl[])
            n329 = Negate(x=w463) -> (-x=w465:dbl[])
            n330 = local read "y_left"() -> (w464:dbl[])
            n331 = Increment(x=w453) -> (x+1=w452:i32)
            n332 = call <vilib>:"General Polynomial Fit Coefficients.vi"("Y"=w465, "polynomial order"=w452, "X"=w464) -> ("Polynomial Coefficients"=w461:dbl[])  [unwired: 11 in, 1 out]
            n333 = Negate(x=w461) -> (-x=w451:dbl[])
            n334 = local read "y_left"() -> (w460:dbl[])
            n335 = call-poly <vilib>:"Polynomial Evaluation.vi"("P(x)"=w451, "A"=w460) -> ("P(A)"=w462:dbl[])  [unwired: 1 out]
            n336 = local read "x_left"() -> (w459:dbl[])
            n337 = Subtract(x=w462, y=w459) -> (x-y=w456:dbl[])
            n338 = Absolute Value(x=w456) -> (abs(x)=w455:dbl[])
            n339 = Add Array Elements(numeric array=w455) -> (sum=w458:dbl)
            n340 = Array Size(array=w455) -> (size(s)=w457:i32)
            n341 = Divide(x=w458, y=w457) -> (x/y=w454:dbl)
          }
          n342 = Multiply(x=w440, y=dbl[] [1.0, 1.1, 1.15]) -> (x*y=w439:dbl[])
          n343 = Array Max & Min(array=w439) -> (min index (indices)=w438:i32)  [unwired: 3 out]
          n344 = Index Array(array=w449, index (row)=w438) -> (element=w435:dbl[])  [unwired: 1 in]
          n345 = Array Subset(array=w435, index=1) -> (w443:dbl[])  [unwired: 1 in]
          n346 = Absolute Value(x=w443) -> (abs(x)=w444:dbl[])
          n347 = Not Equal To 0?(x=w438) -> (x != 0?=w437:bool)
          n348 = Greater?(x=w444, y=1.0) -> (0:w446:bool[])
          n349 = Or Array Elements(Boolean array=w446) -> (logical OR=w447:bool)
          n350 = Select(t=dbl[] [], s=w447, f=w435) -> (s? t:f=w436:dbl[])
          n351 = Select(t=w436, s=w437, f=w435) -> (s? t:f=w434:dbl[])
          n352 = local write "Coeff left"(w434) -> ()
        }
        frame True {
          n353 = local write "Coeff left"(dbl[] []) -> ()
        }
      }
    }
    frame #6 {
      n354 = local read "Coeff right"() -> (w470:dbl[])
      n355 = local read "Coeff left"() -> (w471:dbl[])
      n356 = Empty Array?(array=w471) -> (empty?=w467:bool)
      n357 = Empty Array?(array=w470) -> (empty?=w469:bool)
      n358 = Exclusive Or(1:w469, 2:w467) -> (0:w468:bool)
      n359 = case shown="False" w468 {
        tunnel: w467 -> [_ w496]
        frame False {
          n360 = flat-sequence {
            frame #0 {
              n361 = local read "Coeff right"() -> (w475:dbl[])
              n362 = local read "Coeff left"() -> (w476:dbl[])
              n363 = Index Array(array=w476) -> (element=w474:dbl)  [unwired: 1 in]
              n364 = Index Array(array=w475) -> (element=w473:dbl)  [unwired: 1 in]
              n365 = Greater?(x=w474, y=w473) -> (0:w472:bool)
              n366 = case shown="True" w472 {
                frame False {
                }
                frame True {
                  n367 = flat-sequence {
                    frame #0 {
                      n368 = local read "x_right"() -> (→"x_tmp":dbl[])
                      n369 = local read "Coeff right"() -> (→"c_tmp":dbl[])
                      n370 = local read "y_right"() -> (→"y_tmp":dbl[])
                    }
                    frame #1 {
                      n371 = local read "x_left"() -> (w480:dbl[])
                      n372 = local read "y_left"() -> (w481:dbl[])
                      n373 = local read "Coeff left"() -> (w482:dbl[])
                      n374 = local write "x_right"(w480) -> ()
                      n375 = local write "y_right"(w481) -> ()
                      n376 = local write "Coeff right"(w482) -> ()
                    }
                    frame #2 {
                      n377 = local read "y_tmp"() -> (w484:dbl[])
                      n378 = local read "c_tmp"() -> (w483:dbl[])
                      n379 = local read "x_tmp"() -> (w485:dbl[])
                      n380 = local write "y_left"(w484) -> ()
                      n381 = local write "Coeff left"(w483) -> ()
                      n382 = local write "x_left"(w485) -> ()
                    }
                  }
                }
              }
            }
            frame #1 {
              n383 = local read "Coeff right"() -> (w487:dbl[])
              n384 = local read "Coeff left"() -> (w486:dbl[])
              n385 = local read "Coeff left"() -> (w491:dbl[])
              n386 = Add(x=w486, y=w487) -> (x+y=w495:dbl[])
              n387 = Subtract(x=w487, y=w491) -> (x-y=w490:dbl[])
              n388 = Index Array(array=w490, index=0) -> (element=w488:dbl)
              n389 = Multiply(x=w495, y=0.5) -> (x*y=w493:dbl[])
              n390 = Reverse 1D Array(array=w493) -> (reversed array=w492:dbl[])
              n391 = global write "G_SEN.vi" "vision lane width"(w488) -> ()
              n392 = global write "G_SEN.vi" "Lane_C_M"(w492) -> ()
            }
          }
        }
        frame True {
          n393 = case shown="True" w496 {
            frame False {
              n394 = flat-sequence {
                frame #0 {
                  n395 = local read "Coeff left"() -> (w501:dbl[])
                  n396 = Index Array(array=w501, index=0) -> (element=w499:dbl)
                  n397 = Greater?(x=w499, y=0.5) -> (0:w497:bool)
                  n398 = case shown="True" w497 {
                    frame False {
                    }
                    frame True {
                      n399 = flat-sequence {
                        frame #0 {
                          n400 = local read "y_left"() -> (w503:dbl[])
                          n401 = local read "x_left"() -> (w502:dbl[])
                          n402 = local read "Coeff left"() -> (w504:dbl[])
                          n403 = local write "x_right"(w502) -> ()
                          n404 = local write "y_right"(w503) -> ()
                          n405 = local write "Coeff right"(w504) -> ()
                        }
                        frame #1 {
                          w505 = dbl[] []
                          n406 = local write "y_left"(w505) -> ()
                          n407 = local write "x_left"(w505) -> ()
                          n408 = local write "Coeff left"(w505) -> ()
                        }
                      }
                    }
                  }
                }
                frame #1 {
                  n409 = global read "G_SEN.vi" "vision lane width"() -> (w515:dbl)
                  n410 = local read "Coeff left"() -> (w513:dbl[])
                  n411 = Index Array(array=w513, index=0) -> (element=w511:dbl)
                  n412 = Multiply(x=w515, y=0.5) -> (x*y=w510:dbl)
                  n413 = Add(x=w511, y=w510) -> (x+y=w508:dbl)
                  n414 = Replace Array Subset(array=w513, new element=w508, index=0) -> (w506:dbl[])
                  n415 = Reverse 1D Array(array=w506) -> (reversed array=w509:dbl[])
                  n416 = global write "G_SEN.vi" "Lane_C_M"(w509) -> ()
                }
              }
            }
            frame True {
              n417 = flat-sequence {
                frame #0 {
                  n418 = local read "Coeff right"() -> (w520:dbl[])
                  n419 = Index Array(array=w520, index=0) -> (element=w518:dbl)
                  n420 = Less?(x=w518, y=-0.5) -> (x < y?=w516:bool)
                  n421 = case shown="True" w516 {
                    frame False {
                    }
                    frame True {
                      n422 = flat-sequence {
                        frame #0 {
                          n423 = local read "x_right"() -> (w521:dbl[])
                          n424 = local read "Coeff right"() -> (w523:dbl[])
                          n425 = local read "y_right"() -> (w522:dbl[])
                          n426 = local write "x_left"(w521) -> ()
                          n427 = local write "Coeff left"(w523) -> ()
                          n428 = local write "y_left"(w522) -> ()
                        }
                        frame #1 {
                          w524 = dbl[] []
                          n429 = local write "x_right"(w524) -> ()
                          n430 = local write "y_right"(w524) -> ()
                          n431 = local write "Coeff right"(w524) -> ()
                        }
                      }
                    }
                  }
                }
                frame #1 {
                  n432 = global read "G_SEN.vi" "vision lane width"() -> (w534:dbl)
                  n433 = local read "Coeff right"() -> (w532:dbl[])
                  n434 = Index Array(array=w532, index=0) -> (element=w530:dbl)
                  n435 = Multiply(x=w534, y=0.5) -> (x*y=w529:dbl)
                  n436 = Subtract(x=w530, y=w529) -> (x-y=w527:dbl)
                  n437 = Replace Array Subset(array=w532, new element=w527, index=0) -> (w525:dbl[])
                  n438 = Reverse 1D Array(array=w525) -> (reversed array=w528:dbl[])
                  n439 = global write "G_SEN.vi" "Lane_C_M"(w528) -> ()
                }
              }
            }
          }
        }
      }
    }
    frame #7 {
      n440 = local read "Coeff right"() -> (w535:dbl[])
      n441 = local read "Coeff left"() -> (w536:dbl[])
      n442 = global write "G_SEN.vi" "Lane_R_M"(w535) -> ()
      n443 = global write "G_SEN.vi" "Lane_L_M"(w536) -> ()
    }
    frame #8 {
      n444 = local read "error right"() -> (→"right":dbl[])
      n445 = local read "error left"() -> (→"left":dbl[])
      n446 = local read "y_right"() -> (w549:dbl[])
      n447 = local read "y_left"() -> (w540:dbl[])
      n448 = Array Max & Min(array=w540) -> (max value=w541:dbl, min value=w543:dbl)  [unwired: 2 out]
      n449 = Array Max & Min(array=w549) -> (max value=w548:dbl, min value=w546:dbl)  [unwired: 2 out]
      n450 = Increment(x=w541) -> (x+1=w542:dbl)
      n451 = Decrement(x=w543) -> (x-1=w544:dbl)
      n452 = Increment(x=w548) -> (x+1=w547:dbl)
      n453 = Decrement(x=w546) -> (x-1=w545:dbl)
      n454 = call-poly <vilib>:"Ramp Pattern.vi"("start"=w544, "end"=w542, "delta"=0.01) -> ("Ramp Pattern"=w537:dbl[])  [unwired: 6 in, 2 out]
      n455 = call-poly <vilib>:"Ramp Pattern.vi"("start"=w545, "end"=w547, "delta"=0.01) -> ("Ramp Pattern"=w538:dbl[])  [unwired: 6 in, 2 out]
      n456 = local read "Coeff right"() -> (w558:dbl[])
      n457 = local read "Coeff left"() -> (w562:dbl[])
      n458 = local read "y origin"() -> (w574:dbl[])
      n459 = local read "y_right"() -> (w555:dbl[])
      n460 = local read "y_left"() -> (w560:dbl[])
      n461 = local read "x origin"() -> (w572:dbl[])
      n462 = local read "x_right"() -> (w559:dbl[])
      n463 = local read "x_left"() -> (w561:dbl[])
      n464 = call-poly <vilib>:"Polynomial Evaluation.vi"("P(x)"=w562, "A"=w537) -> ("P(A)"=w570:dbl[])  [unwired: 1 out]
      n465 = call-poly <vilib>:"Polynomial Evaluation.vi"("P(x)"=w558, "A"=w538) -> ("P(A)"=w571:dbl[])  [unwired: 1 out]
      n466 = call "Convert to Dynamic Data"("Array"=w537) -> ("Dynamic Data Type"=w568:dynamicdata)  [unwired: 3 in]
      n467 = call "Convert to Dynamic Data7"("Array"=w538) -> ("Dynamic Data Type"=w554:dynamicdata)  [unwired: 3 in]
      n468 = call "Convert to Dynamic Data3"("Array"=w560) -> ("Dynamic Data Type"=w563:dynamicdata)  [unwired: 3 in]
      n469 = call "Convert to Dynamic Data8"("Array"=w555) -> ("Dynamic Data Type"=w553:dynamicdata)  [unwired: 3 in]
      n470 = call "Convert to Dynamic Data10"("Array"=w574) -> ("Dynamic Data Type"=w575:dynamicdata)  [unwired: 3 in]
      n471 = call "Convert to Dynamic Data2"("Array"=w570) -> ("Dynamic Data Type"=w567:dynamicdata)  [unwired: 3 in]
      n472 = call "Convert to Dynamic Data4"("Array"=w561) -> ("Dynamic Data Type"=w565:dynamicdata)  [unwired: 3 in]
      n473 = call "Convert to Dynamic Data5"("Array"=w571) -> ("Dynamic Data Type"=w557:dynamicdata)  [unwired: 3 in]
      n474 = call "Convert to Dynamic Data6"("Array"=w559) -> ("Dynamic Data Type"=w556:dynamicdata)  [unwired: 3 in]
      n475 = call "Convert to Dynamic Data9"("Array"=w572) -> ("Dynamic Data Type"=w573:dynamicdata)  [unwired: 3 in]
      n476 = Merge Signals(w568, w563, w554, w553, w575) -> (w564:dynamicdata)
      n477 = Merge Signals(w567, w565, w557, w556, w573) -> (w566:dynamicdata)
      n478 = call "Build XY Graph"("Y Input"=w564, "X Input"=w566) -> ("XY Graph"=→"XY Graph 4":cluster{"X":dbl[], "Y":dbl[]}[])  [unwired: 8 in, 1 out]
    }
  }
